vi "ScrapAnalyzerEnergy.vi"() -> ()   [LabVIEW 2014]
panel:
  out "Number of Steps":i32
  out "BraggArray":dbl[](array[numeric])
  in  "EnergyStep":dbl
  in  "Energy Range":cluster{dbl, dbl}(slide)={0.0, 5.858585858585858} scale=9633.510566263154..10202.103959256357
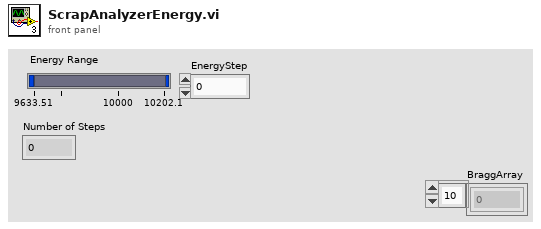
[diagram p1: front panel]
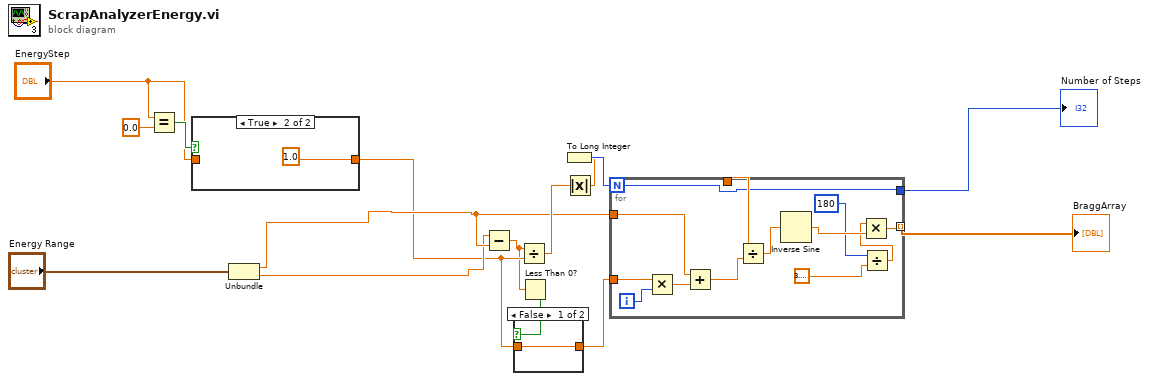
[diagram p0: block diagram]
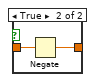
[diagram p2: hidden frame]
diagram:
  n1 = Equal?(x="EnergyStep", y=0.0) -> (x = y?=w10:bool)
  n2 = case shown="True" w10 {
    tunnel: "EnergyStep" -> [w16 _]
    tunnel: [w16 1.0] -> w4
    frame False {
    }
    frame True {
    }
  }
  n3 = Unbundle("Energy Range") -> (w12:dbl, w11:dbl)
  n4 = Subtract(x=w11, y=w12) -> (x-y=w3:dbl)
  n5 = Divide(x=w3, y=w4) -> (x/y=w14:dbl)
  n6 = Less Than 0?(x=w3) -> (x < 0?=w6:bool)
  n7 = case shown="False" w6 {
    tunnel: [w18 w20] -> w5
    tunnel: w4 -> [w18 w19]
    frame False {
    }
    frame True {
      n8 = Negate(x=w19) -> (-x=w20:dbl)
    }
  }
  n9 = Absolute Value(x=w14) -> (abs(x)=w1:dbl)
  n10 = To Long Integer(number=w1) -> (32bit integer=w2:i32)
  n11 = for {
    N: w2 -> [w24]
    tunnel: w12 -> [w31]
    tunnel: [w23] -> w15 mode=indexing
    tunnel: w5 -> [w26]
    tunnel: _ -> [w25]
    tunnel: [w24] -> w7
    i -> [w33]
    n12 = Multiply(x=w26, y=w33) -> (x*y=w32:dbl)
    n13 = Add(x=w31, y=w32) -> (x+y=w30:dbl)
    n14 = Divide(x=w25, y=w30) -> (x/y=w29:dbl)
    n15 = Inverse Sine(1:w29) -> (0:w28:dbl)
    n16 = Divide(x=180, y=3.141592653589793) -> (x/y=w22:dbl)
    n17 = Multiply(x=w22, y=w28) -> (x*y=w23:dbl)
  }
  "BraggArray" <- w15
  "Number of Steps" <- w7
